vi "Update Annotations.vi"(6 "Sample Period":dbl, 8 "Commands":cluster{"Time (s)":dbl, T3, "Enabled":bool}[](array[cluster]), 9 "TrajDataIn":T2(array[cluster]), 10 "Robot Pt Index":i32, 11 "dt array":dbl[](array[numeric])) -> (1 "Redraw":bool, 2 "Velocity Trace":dbl[](array[numeric]), 3 "Annotation Data":T5(array[cluster]))   [LabVIEW 2025]
uses:
  Types/Single Cmd Info.ctl
  <vilib>/picture/picture.llb/imagedata.ctl
  Types/Segment Type.ctl
panel:
  out "Array":dbl[](array[numeric])
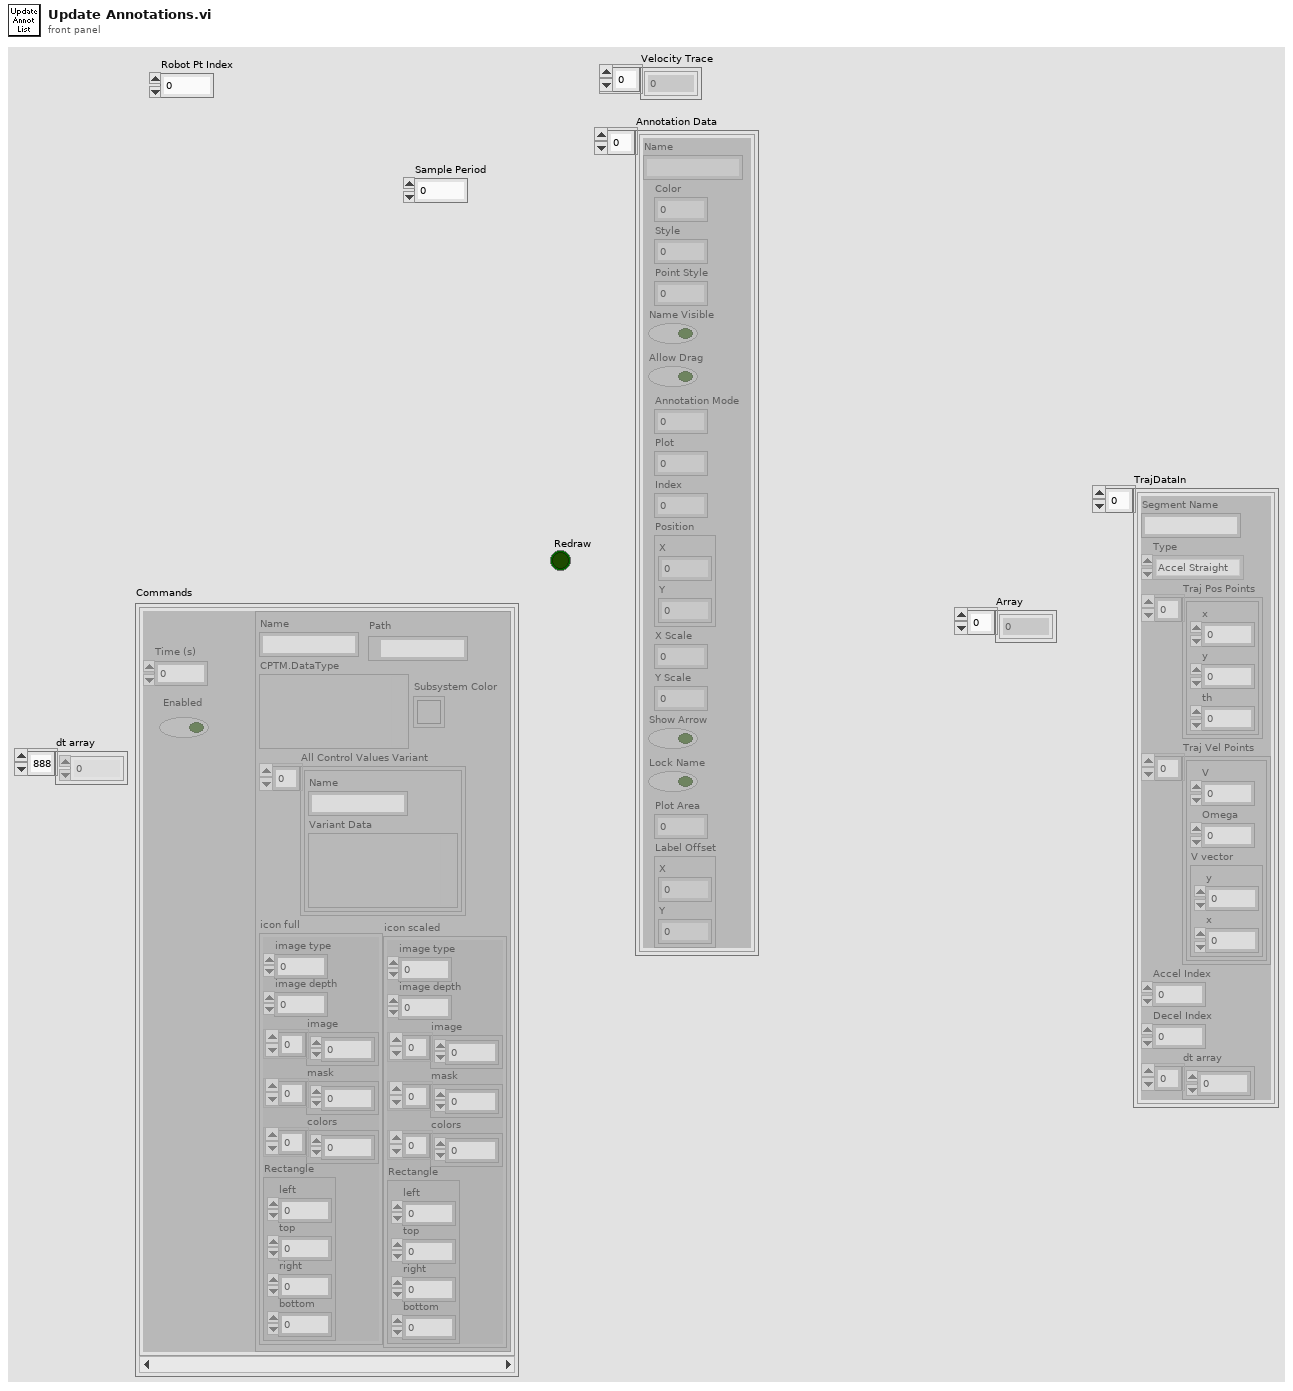
[diagram p1: front panel]
types:
  T1 = typedef "Segment Type.ctl" = enum16{"Accel Straight", "Const Straight", "Blend", "Circle", "Bezier", "Choreo"}
  T2 = cluster{"Segment Name":string, "Type":T1, "Traj Pos Points":cluster{"x":dbl, "y":dbl, "th":dbl}[], "Traj Vel Points":cluster{"V":dbl, "Omega":dbl, "V vector":cluster{"y":dbl, "x":dbl}}[], "Accel Index":i32, "Decel Index":i32, "dt array":dbl[]}[]
  T3 = typedef "Single Cmd Info.ctl" = cluster{"Name":string, "CPTM.DataType":variant, "All Control Values Variant":cluster{"Name":string, "Variant Data":variant}[], "icon full":T4, "icon scaled":T4, "Path":path, "Subsystem Color":u32}
  T4 = typedef "imagedata.ctl" = cluster{"image type":i32, "image depth":i32, "image":u8[], "mask":u8[], "colors":u32[], "Rectangle":cluster{"left":i16, "top":i16, "right":i16, "bottom":i16}}
  T5 = cluster{"Name":string, "Color":u32, "Style":i32, "Point Style":i32, "Name Visible":bool, "Allow Drag":bool, "Annotation Mode":i32, "Plot":i32, "Index":i32, "Position":cluster{"X":dbl, "Y":dbl}, "X Scale":i32, "Y Scale":u32, "Show Arrow":bool, "Lock Name":bool, "Plot Area":i32, "Label Offset":cluster{"X":dbl, "Y":dbl}}[]
  T6 = cluster{"Name":string, "Color":u32, "Style":i32, "Point Style":i32, "Name Visible":bool, "Allow Drag":bool, "Annotation Mode":i32, "Plot":i32, "Index":i32, "Position":cluster{"X":dbl, "Y":dbl}, "X Scale":i32, "Y Scale":u32, "Show Arrow":bool, "Lock Name":bool, "Plot Area":i32, "Label Offset":cluster{"X":dbl, "Y":i32}}
  T7 = enum16{"Accel Straight", "Const Straight", "Blend", "Circle"}
  T8 = cluster{"V":dbl, "Omega":dbl, "V vector":cluster{"y":dbl, "x":dbl}}[]
  T9 = cluster{"Name":string, "Color":u32, "Style":i32, "Point Style":i32, "Name Visible":bool, "Allow Drag":bool, "Annotation Mode":i32, "Plot":i32, "Index":i32, "Position":cluster{"X":dbl, "Y":dbl}, "X Scale":i32, "Y Scale":u32, "Show Arrow":bool, "Lock Name":bool, "Plot Area":i32, "Label Offset":cluster{"X":dbl, "Y":i32}}[]
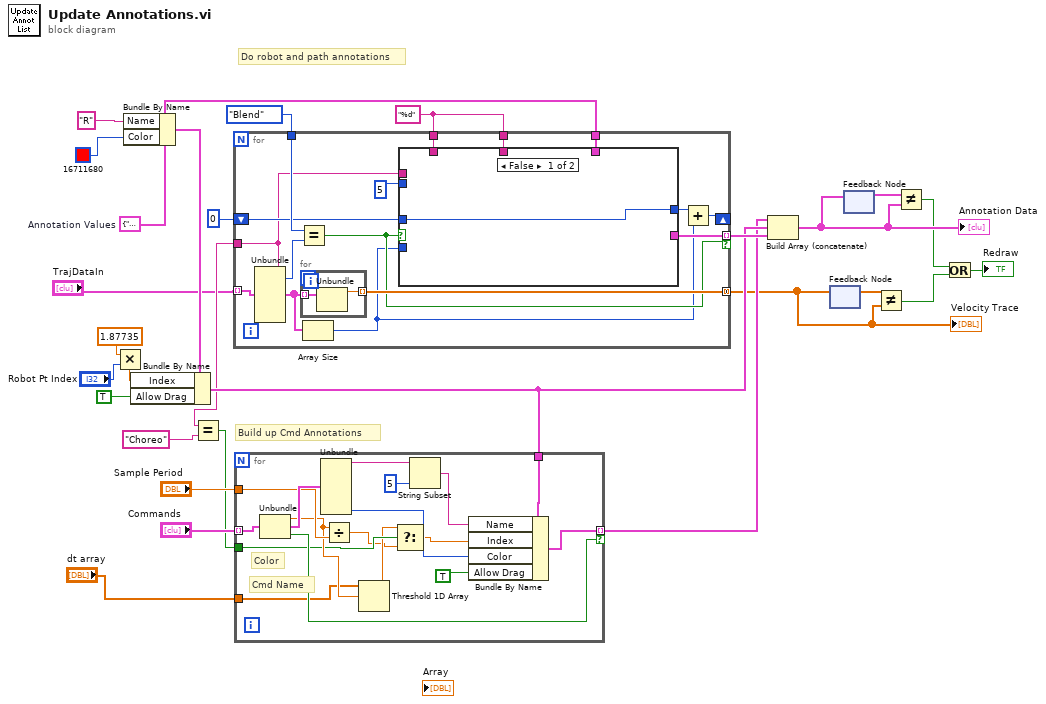
[diagram p0: block diagram]
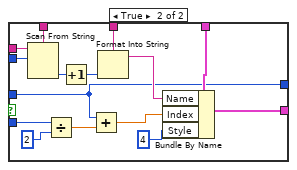
[diagram p2: hidden frame]
diagram:
  w21 = T6 {"Name"="", "Color"=16776608, "Style"=5, "Point Style"=3, "Name Visible"=TRUE, "Allow Drag"=FALSE, "Annotation Mode"=1, "Plot"=0, "Index"=0, "Position"={"X"=0.0, "Y"=0.0}, "X Scale"=0, "Y Scale"=0, "Show Arrow"=FALSE, "Lock Name"=FALSE, "Plot Area"=0, "Label Offset"={"X"=0.6, "Y"=-2}}  # Annotation Values
  w24 = "%d" ("Name")
  # "Do robot and path annotations"
  # "Build up Cmd Annotations"
  n1 = Multiply(x=1.87735, y="Robot Pt Index") -> (x*y=w2:dbl)
  n2 = Bundle By Name(cluster=w21, "Name"="R", "Color"=u32 16711680) -> (w28:T6)
  n3 = Bundle By Name(cluster=w28, "Index"=w2, "Allow Drag"=TRUE ("Name Visible")) -> (w18:T6)
  n4 = for {
    tunnel: "TrajDataIn" -> [w44] mode=indexing
    tunnel: [w43] -> w12 mode=concatenating
    tunnel: T7."Blend" ("Type") -> [w42]
    shift-right: [w32] -> _
    shift-left: 0 -> [w39]
    tunnel: [w35] -> w25 mode=indexing if=w34
    tunnel: w21 -> [w38]
    tunnel: w24 -> [w37]
    tunnel: w24 -> [w36]
    tunnel: [w29] -> w7
    n5 = Unbundle(w44) -> ("Segment Name"=w29:string, "Type"=w41:T1, "Traj Vel Points"=w40:T8)  [unwired: 4 out]
    n6 = Equal?(x=w42, y=w41) -> (x = y?=w34:bool)
    n7 = for {
      tunnel: w40 -> [w62] mode=indexing
      tunnel: [w61] -> w43 mode=indexing
      n8 = Unbundle(w62) -> ("V"=w61:dbl)  [unwired: 2 out]
    }
    n9 = Array Size(array=w40) -> (size(s)=w31:i32)
    n10 = case shown="False" w34 {
      tunnel: w39 -> [w45 w54]
      tunnel: [w45 w54] -> w33
      tunnel: w38 -> [_ w60]
      tunnel: w29 -> [_ w59]
      tunnel: w37 -> [_ w58]
      tunnel: w36 -> [_ w57]
      tunnel: [_ w55] -> w35
      tunnel: w31 -> [_ w51]
      tunnel: 5 -> [_ w50]
      frame False {
      }
      frame True {
        n11 = Scan From String(format string=w58, input string=w59, initial scan location=w50) -> (output 1=w48:i32)  [unwired: 2 in, 3 out]
        n12 = Divide(x=w51, y=2) -> (x/y=w52:dbl)
        n13 = Increment(x=w48) -> (x+1=w47:i32)
        n14 = Add(x=w54, y=w52) -> (x+y=w49:dbl)
        n15 = Format Into String(format string=w57, w47) -> (resulting string=w56:string)  [unwired: 2 in, 1 out]
        n16 = Bundle By Name(cluster=w60, "Name"=w56, "Index"=w49, "Style"=4) -> (w55:T6)
      }
    }
    n17 = Add(x=w33, y=w31) -> (x+y=w32:i32)
  }
  "Velocity Trace" <- w12
  n18 = Equal?(x=w7, y="Choreo") -> (x = y?=w5:bool)
  n19 = for {
    tunnel: "Commands" -> [w79] mode=indexing
    tunnel: w18 -> [w78]
    tunnel: [w77] -> w17 mode=indexing if=w74
    tunnel: "Sample Period" -> [w69]
    tunnel: "dt array" -> [w67]
    tunnel: w5 -> [w66]
    # "Cmd Name"
    # "Color"
    n20 = Unbundle(w79) -> ("Time (s)"=w68:dbl, w75:T3, "Enabled"=w74:bool)
    n21 = Unbundle(w75) -> ("Name"=w73:string, "Subsystem Color"=w70:u32)  [unwired: 5 out]
    n22 = Divide(x=w68, y=w69) -> (x/y=w64:dbl)
    n23 = Threshold 1D Array(2:w68, 3:w67) -> (0:w65:dbl)  [unwired: 1 in]
    n24 = Select(t=w65, s=w66, f=w64) -> (s? t:f=w63:dbl)
    n25 = String Subset(string=w73, length (rest)=5 ("length (rest)")) -> (substring=w71:string)  [unwired: 1 in]
    n26 = Bundle By Name(cluster=w78, "Name"=w71, "Index"=w63, "Color"=w70, "Allow Drag"=TRUE ("Name Visible")) -> (w77:T6)
  }
  n27 = Build Array (concatenate)(w17, w18, w25) -> (w14:T9)
  "Annotation Data" <- w14
  n28 = feedback #1() -> (w13:dbl[])  [unwired: 1 in]
  n29 = feedback-in #1(w12) -> ()
  n30 = feedback-in #2(w14) -> ()
  n31 = feedback #2() -> (w15:T9)  [unwired: 1 in]
  n32 = Not Equal?(x=w13, y=w12) -> (x != y?=w10:bool)
  n33 = Not Equal?(x=w15, y=w14) -> (x != y?=w11:bool)
  n34 = Or(x=w11, y=w10) -> (x .or. y?=→"Redraw":bool)
